vi "P3060_根据槽位打开设备.vi"(8 "error in (no error)":errorcluster caption="错误输入（无错误）", 10 "机箱号":i16=1, 11 "槽位号":i16) -> (0 "error out":errorcluster caption="错误输出", 3 "句柄输出":i32)   [LabVIEW 2012]
doc: "打开板卡操作，输出板卡句柄！当有多个板卡时，根据板卡索引号打开不同板卡！\n如果同时使用一块板卡的多种功能，可将输出句柄连接到不同的功能任务中。\n此VI是创建所有任务的前提！"
uses:
  _SubVI/dll/Release/P3060.dll
panel:
  out "return":i32
  out "错误输出":errorcluster
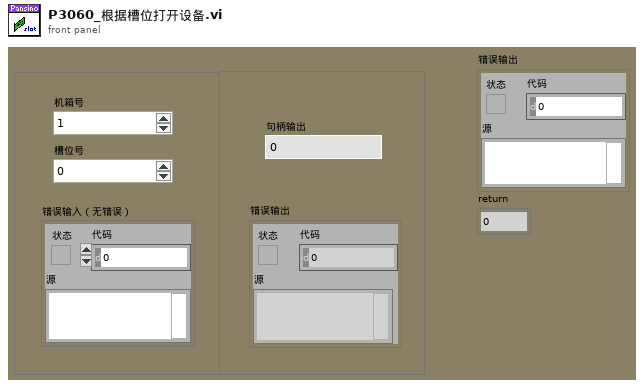
[diagram p1: front panel]
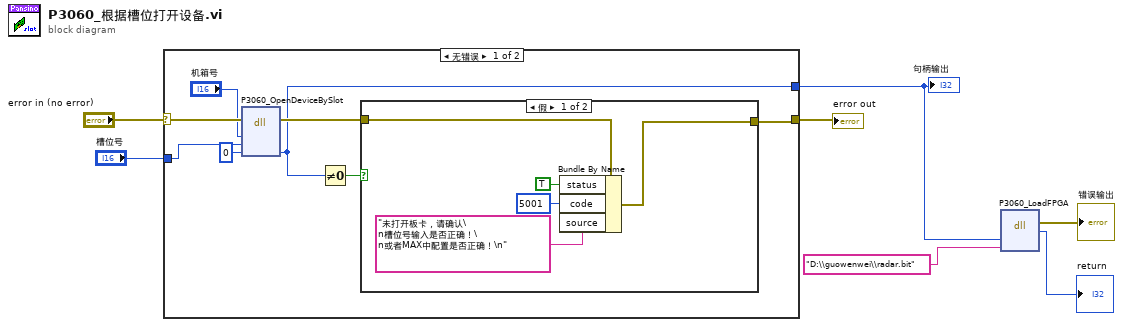
[diagram p0: block diagram]
diagram:
  n1 = case shown="无错误" "error in (no error)" {
    selector: "error in (no error)" -> [w15 w22]
    tunnel: [w11 w22] -> w5
    tunnel: "槽位号" -> [w14 _]
    tunnel: [w10 _] -> w4
    frame No Error {
      n2 = dll-call lib="C:/PLC_simulation/2014.2.25PLC_NEW/PLC_NEW/P3060NEW/_SubVI/dll/Release/P3060.dll" fn="P3060_OpenDeviceBySlot"(error in=w15, "Classis"="机箱号", "槽位号"=w14, "设备句柄"=0) -> (error out=w12:errorcluster, "设备句柄"=w10:i32)  [unwired: 5 in, 1 out]
      n3 = Not Equal To 0?(x=w10) -> (x != 0?=w13:bool)
      n4 = case shown="假" w13 {
        tunnel: w12 -> [w20 w21]
        tunnel: [w16 w21] -> w11
        frame False {
          n5 = Bundle By Name(cluster=w20, "status"=TRUE, "code"=5001, "source"="未打开板卡，请确认\n槽位号输入是否正确！\n或者MAX中配置是否正确！\n") -> (w16:errorcluster)
        }
        frame True {
        }
      }
    }
    frame Error {
    }
  }
  "句柄输出" <- w4
  "error out" <- w5
  n6 = dll-call lib="C:/PLC_simulation/2014.2.25PLC_NEW/PLC_NEW/P3060NEW/_SubVI/dll/Release/P3060.dll" fn="P3060_LoadFPGA"("hDev"=w4, "filepath"="D:\\guowenwei\\radar.bit") -> (error out=→"错误输出":errorcluster, "return"=→"return":i32)  [unwired: 5 in, 1 out]
